vi "FTW-ProjectItem-Tag-GetVariant.vi"(0 "ProjectItem":refnum<vi>, 5 "Tag Name":string, 11 "error in":errorcluster) -> (4 "ProjectItem out":refnum<vi>, 6 "Tag Value":variant, 8 "Persistent?":bool, 10 "Exists?":bool, 15 "error out":errorcluster)   [LabVIEW 2012]
panel:
  # "Inputs"
  # "Outputs"
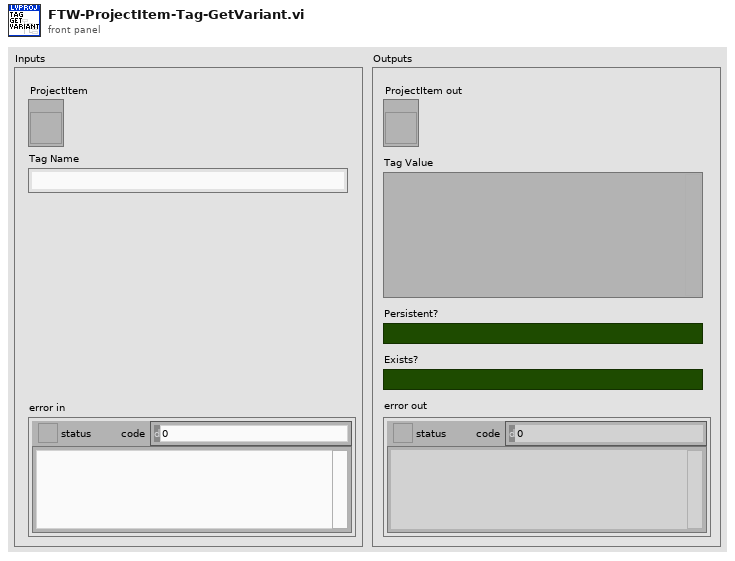
[diagram p1: front panel]
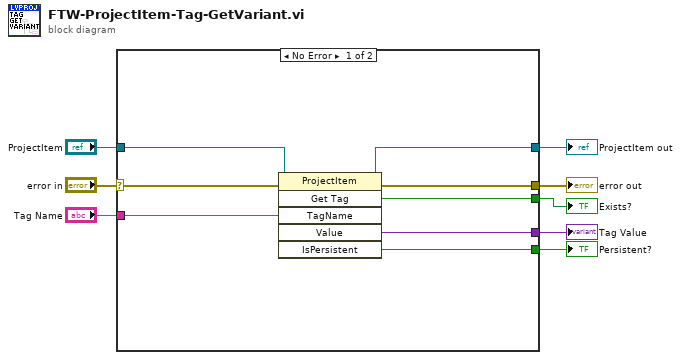
[diagram p0: block diagram]
diagram:
  n1 = case shown="No Error" "error in" {
    selector: "error in" -> [w16 w18]
    tunnel: [w15 w18] -> w8
    tunnel: "Tag Name" -> [w14 _]
    tunnel: "ProjectItem" -> [w13 w17]
    tunnel: [w12 w17] -> w4
    tunnel: [w11 _] -> w3
    tunnel: [w10 _] -> w2
    tunnel: [w9 _] -> w1
    frame No Error {
      n2 = invoke class="ProjectItem" method="Get Tag"(reference=w13, error in=w16, "TagName"=w14) -> (reference out=w12:refnum<vi>, error out=w15:errorcluster, "GetTag"=w11:bool, "Value"=w10:variant, "IsPersistent"=w9:bool)  [unwired: 3 in, 1 out]
    }
    frame Error {
    }
  }
  "error out" <- w8
  "Tag Value" <- w2
  "Persistent?" <- w1
  "ProjectItem out" <- w4
  "Exists?" <- w3
